vi "Send Data Message.vi"(8 "error in (no error)":errorcluster, 10 "Message":string, 11 "WebSocket in":refnum<class "WebSocket.lvclass">) -> (0 "error out":errorcluster, 3 "WebSocket out":refnum<class "WebSocket.lvclass">)   [LabVIEW 2023, in "WebSocket.lvclass"]
uses:
  WebSocket.lvclass
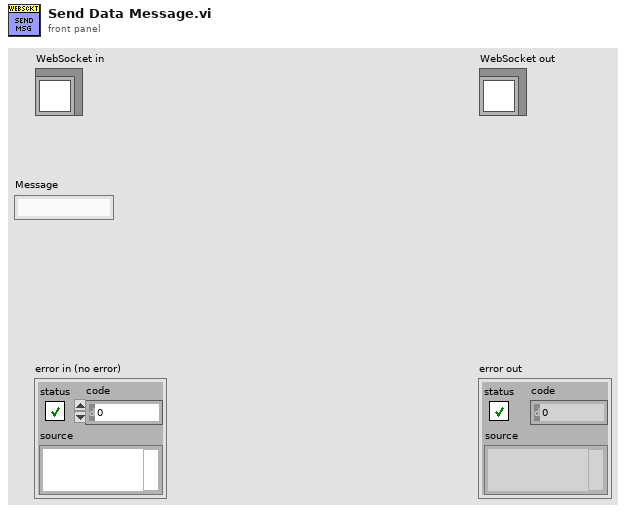
[diagram p1: front panel]
types:
  T1 = typedef "WebSocket.lvclass/ObjectAttributes.ctl" = cluster{"Socket":refnum<k5>, "Thread":refnum<vi>, "From Socket":refnum<queue>, "To Socket":refnum<queue>, "Rx Stats in Progress":variant, "Rx Stats":variant, "Tx Stats in Progress":variant, "Tx Stats":variant}
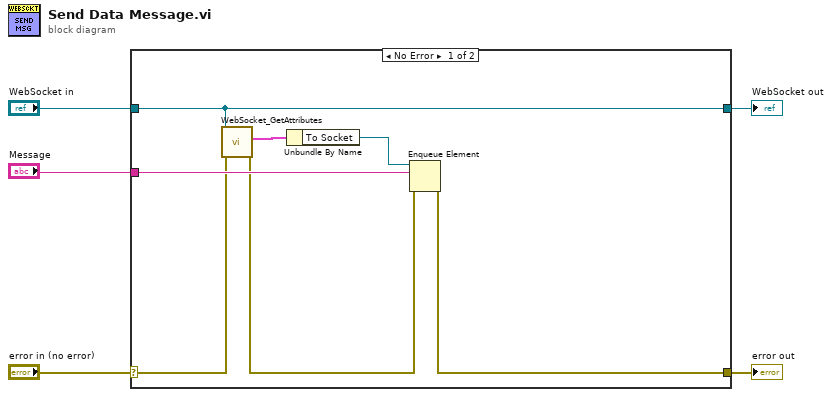
[diagram p0: block diagram]
diagram:
  n1 = case shown="No Error" "error in (no error)" {
    selector: "error in (no error)" -> [w7 w14]
    tunnel: [w10 w14] -> w4
    tunnel: [w9 w13] -> w2
    tunnel: "WebSocket in" -> [w9 w13]
    tunnel: "Message" -> [w11 _]
    frame No Error {
      n2 = call "WebSocket_GetAttributes.vi"("error in (no error)"=w7, "reference in"=w9) -> ("error out"=w6:errorcluster, "Data"=w8:T1)  [unwired: 6 in, 2 out]
      n3 = Unbundle By Name(w8) -> ("To Socket"=w12:refnum<queue>)
      n4 = Enqueue Element(queue=w12, element=w11, error in (no error)=w6) -> (error out=w10:errorcluster)  [unwired: 1 in, 2 out]
    }
    frame Error {
    }
  }
  "error out" <- w4
  "WebSocket out" <- w2
